vi "cluster_to_1darray_withscaling.vi"(7 "scaling":dbl=1.0 format="%#_13g", 10 "B":cluster{"Bx":dbl[], "By":dbl[], "Bz":dbl[]}) -> (2 "scaledBarray":dbl[](array[numeric]))   [LabVIEW 2017]
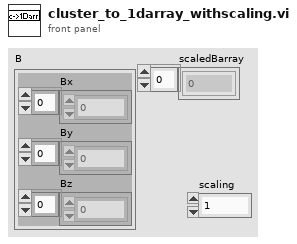
[diagram p1: front panel]
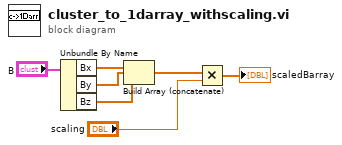
[diagram p0: block diagram]
diagram:
  n1 = Unbundle By Name("B") -> ("Bx"=w6:dbl[], "By"=w5:dbl[], "Bz"=w4:dbl[])
  n2 = Build Array (concatenate)(w6, w5, w4) -> (w3:dbl[])
  n3 = Multiply(x=w3, y="scaling") -> (x*y=→"scaledBarray":dbl[])
